vi "ReadSystemDefinitionOverrideFile.vi"(8 "error in (no error)":errorcluster, 11 "configuration file path":path) -> (0 "error out":errorcluster, 2 "properties":T1[](array[typedef]), 3 "overrides":T2[](array[typedef]))   [LabVIEW 2027, in "VeriStandTestUtilities.lvlib"]
uses:
  VeriStandTestUtilities.lvlib
  ConfigOverrideItem.ctl
  ConfigPropertyItem.ctl
  <vilib>/Utility/config.llb/Read Key (String).vi
  <vilib>/regexp/Match Regular Expression.xnode
  <vilib>/Utility/config.llb/NI_LVConfig.lvlib
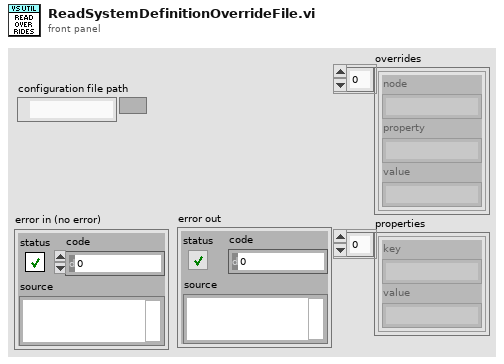
[diagram p1: front panel]
types:
  T1 = typedef "VeriStandTestUtilities.lvlib/ConfigPropertyItem.ctl" = cluster{"key":string, "value":string}
  T2 = typedef "VeriStandTestUtilities.lvlib/ConfigOverrideItem.ctl" = cluster{"node":string, "property":string, "value":string}
  T3 = typedef "NI_LVConfig.lvlib/Config Data RefNum.ctl" = refnum<k1>
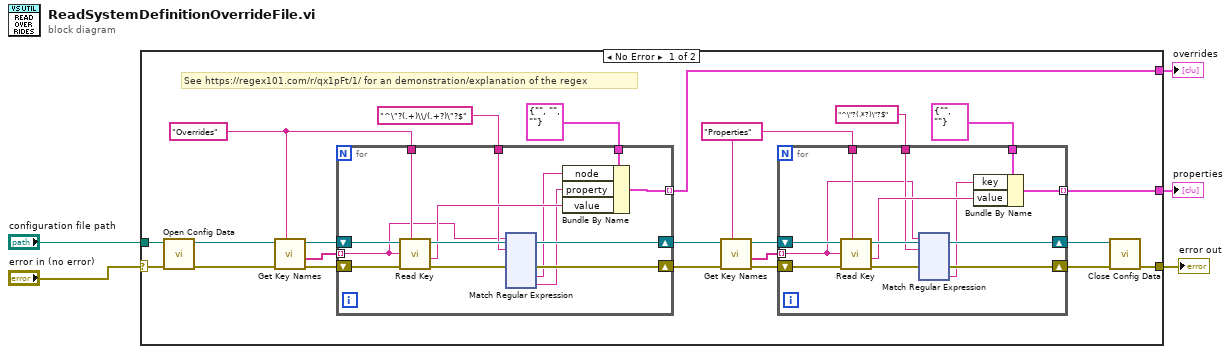
[diagram p0: block diagram]
diagram:
  n1 = case shown="No Error" "error in (no error)" {
    selector: "error in (no error)" -> [w26 w293]
    tunnel: [w28 w293] -> w5
    tunnel: "configuration file path" -> [w27 _]
    tunnel: [w18 _] -> w2
    tunnel: [w7 _] -> w1
    frame No Error {
      w9 = "Properties" ("section")
      w20 = "Overrides" ("section")
      # "See https://regex101.com/r/qx1pFt/1/ for an demonstration/explanation of the regex"
      n2 = call <vilib>:"Open Config Data.vi"("error in (no error)"=w26, "configuration file path"=w27) -> ("error out"=w24:errorcluster, "refnum"=w25:T3)  [unwired: 7 in, 1 out]
      n3 = call <vilib>:"Get Key Names.vi"("section"=w20, "error in (no error)"=w24, "refnum"=w25) -> ("error out"=w23:errorcluster, "key names"=w21:string[], "refnum out"=w22:T3)  [unwired: 5 in, 1 out]
      n4 = for {
        shift-right: [w164] -> w13
        shift-left: w23 -> [w171]
        shift-right: [w170] -> w14
        shift-left: w22 -> [w172]
        tunnel: w21 -> [w160] mode=indexing
        tunnel: w20 -> [w169]
        tunnel: [w167] -> w18 mode=indexing
        tunnel: T2 {"node"="", "property"="", "value"=""} ("override item") -> [w166]
        tunnel: "^\"?(.+)\\/(.+?)\"?$" ("regular expression") -> [w163]
        n5 = call-poly <vilib>:"Read Key.vi"("section"=w169, "error in (no error)"=w171, "key"=w160, "refnum"=w172) -> ("error out"=w165:errorcluster, "value"=w168:string, "refnum out"=w170:T3)  [unwired: 4 in, 1 out]
        n6 = xnode "Match Regular Expression"("input string"=w160, "regular expression"=w163, "error in"=w165) -> ("error out"=w164:errorcluster, "submatch 1"=w162:string, "submatch 2"=w161:string)  [unwired: 3 in, 4 out]
        n7 = Bundle By Name(cluster=w166, "node"=w162, "property"=w161, "value"=w168) -> (w167:T2)
      }
      n8 = call <vilib>:"Get Key Names.vi"("section"=w9, "error in (no error)"=w13, "refnum"=w14) -> ("error out"=w12:errorcluster, "key names"=w10:string[], "refnum out"=w11:T3)  [unwired: 5 in, 1 out]
      n9 = for {
        shift-right: [w32] -> w15
        shift-left: w12 -> [w39]
        shift-right: [w38] -> w16
        shift-left: w11 -> [w40]
        tunnel: w10 -> [w30] mode=indexing
        tunnel: w9 -> [w37]
        tunnel: [w35] -> w7 mode=indexing
        tunnel: T1 {"key"="", "value"=""} ("override item") -> [w36]
        tunnel: "^\"?(.*?)\"?$" ("regular expression") -> [w31]
        n10 = call-poly <vilib>:"Read Key.vi"("section"=w37, "error in (no error)"=w39, "key"=w30, "refnum"=w40) -> ("error out"=w33:errorcluster, "value"=w34:string, "refnum out"=w38:T3)  [unwired: 4 in, 1 out]
        n11 = xnode "Match Regular Expression"("input string"=w30, "regular expression"=w31, "error in"=w33) -> ("error out"=w32:errorcluster, "submatch 1"=w29:string)  [unwired: 3 in, 4 out]
        n12 = Bundle By Name(cluster=w36, "key"=w29, "value"=w34) -> (w35:T1)
      }
      n13 = call <vilib>:"Close Config Data.vi"("error in (no error)"=w15, "refnum"=w16) -> ("error out"=w28:errorcluster)  [unwired: 8 in, 1 out]
    }
    frame Error {
    }
  }
  "error out" <- w5
  "overrides" <- w2
  "properties" <- w1
